vi "Engine-RPC-Sync-B-PID-Host.vi"() -> ()   [LabVIEW 2016]
uses:
  <vilib>/addons/Software Calibration Management/XControls/TBL2D.xctl
panel:
  in  "_ModeTab":T1(tab)
  out "Sync-B_Dur_TdOut":sgl(slide) caption="Dur_ Td Action" max=0 scale=0.0..100.0 scale format="%#.2f"
  out "Sync-B_Dur_TiOut":sgl(slide) caption="Dur_ Ti Action" max=0 scale=0.0..100.0 scale format="%#.2f"
  out "Sync-B_Dur_KpOut":sgl(slide) caption="Dur_ Kc Action" max=0 scale=0.0..100.0 scale format="%#.2f"
  in  "Sync-B_Dur_PIDMin":sgl caption="[%]" format="%#.2f"
  in  "Sync-B_Dur_PIDMax":sgl caption="[%]" max=50 format="%#.2f"
  in  "Sync-B_Dur_Td":sgl caption="[]" format="%#.2f"
  in  "Sync-B_Dur_Ti":sgl caption="[]" format="%#.2f"
  in  "Sync-B_Dur_Kp":sgl caption="[%/bar]" format="%#.2f"
  out "Sync-B_FlowCal_TblOut":sgl caption="[]" format="%#.2f"
  out "Sync-B_DurPID_Out":sgl caption="[%]" max=50
  in  "Sync-B_Dur_NonPIDFF":sgl caption="[]" format="%#.2f"
  out "Sync-B_FuelQty":sgl caption="[mm3/stroke]" format="%#.2f"
  out "Sync-B_PerLobeQty":sgl caption="[mm3/stroke]" format="%#.2f"
  in  "Sync-B_FlowCal_Tbl":cluster{"X":sgl[], "Y":sgl[], "Z":sgl[][]}(xcontrol) caption="[bar|mm3/stroke|ms]"
  # "+"
  # "OR"
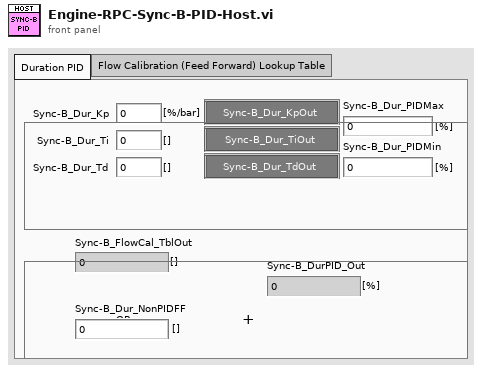
[diagram p1: front panel]
types:
  T1 = enum32{"Duration PID", "Flow Calibration (Feed Forward) Lookup Table"}
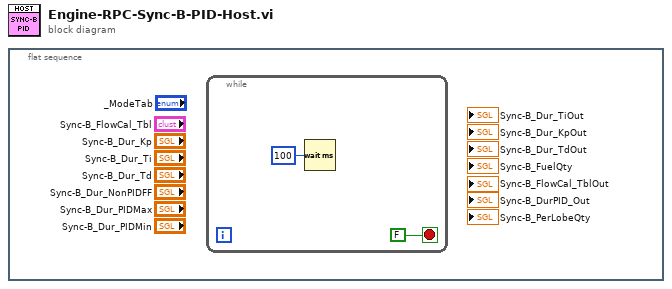
[diagram p0: block diagram]
diagram:
  n1 = flat-sequence {
    frame #0 {
      n2 = while {
        stop <- FALSE stop-if-true
        n3 = Wait (ms)(milliseconds to wait=u32 100) -> ()  [unwired: 1 out]
      }
    }
  }
